vi "Main WT1600 v2.vi"(0 "Settings WT1600 ing":T3={"data bits"=8, "parity"=0, "stop bits"=10, "flow control"=0, "baud rate"=8, "COM"=""} {"baud rate" min=5 max=8 step=1; "flow control" items=["None"=0, "XON/XOFF"=1, "RTS/CTS"=2, "DTR/DSR"=4]; "stop bits" items=["1.0"=10, "1.5"=15, "2.0"=20]; "parity" items=["None", "Odd", "Even", "Mark", "Space"]; "data bits" min=5 max=8 step=1}, 1 "STOP":bool, 2 "Range Tors.":bool, 3 "Numeric":i64, 4 "WT1600 configuration":T2={"Wiring A (0: 1P2W)"=0, "Wiring B (0: 1P2W)"=0, "Wiring C (0: 1P2W)"=0, "V Range (12: 1000)"=12, "Element (0: All)"=0, "Element (0: All) 2"=0, "A Range (9: 5A)"=9, "A Sensor Ratio(mV/A) (10.0000) "=10.0, "Zero Cross Filter (0: OFF)"=0, "Line Filter (0: OFF)"=0, "PT Ratio (1.0000)"=1.0, "Scaling (F: OFF)"=FALSE, "CT Ratio (1.0000)"=1.0, "Scaling Factor (1.0000)"=1.0, "Element (0: All) 3"=0, "Display Format (0: Numeric)"=0, "Normal Item Amount (1: 4)"=1, "Harmonics Item Amount (1: 4)"=1, "Average Type (0: OFF)"=0, "Average Count (2: 8)"=2} {"Average Count (2: 8)" items=["2", "4", "8", "16", "32", "64", "128", "256"]; "Average Type (0: OFF)" items=["OFF", "Linear", "Exponent"]; "Harmonics Item Amount (1: 4)" items=["-", "4", "8", "16", "Single List", "Dual List", "Sigma List"]; "Normal Item Amount (1: 4)" items=["ALL", "4", "8", "16", "42", "78"]; "Display Format (0: Numeric)" items=["Numeric", "Wave", "Bar", "Vector", "Trend", "Numeric & Wave", "Numeric & Bar", "Numeric & Trend", "Wave & Bar", "Wave & Trend", "Bar & Trend", "Information"]; "Element (0: All) 3" items=["All", "Element 1", "Element 2", "Element 3", "Element 4", "Element 5", "Element 6"]; "Scaling Factor (1.0000)" min=0.0001 max=99999.9999 step=0.0001 format="%.4f"; "CT Ratio (1.0000)" min=0.0001 max=99999.9999 step=0.0001 format="%.4f"; "PT Ratio (1.0000)" min=0.0001 max=99999.9999 step=0.0001 format="%.4f"; "Line Filter (0: OFF)" items=["OFF", "500Hz", "5.5kHz"]; "Zero Cross Filter (0: OFF)" items=["OFF", "500Hz"]; "A Sensor Ratio(mV/A) (10.0000)" min=0.0001 max=99999.9999 step=0.0001 format="%.4f"; "A Range (9: 5A)" items=["AUTO", "10 mA", "20 mA", "50 mA", "100 mA", "200 mA", "500 mA", "1 A", "2 A", "5 A", "10 A", "20 A", "50 A", "S-AUTO", "50 mV", "100 mV", "250 mV", "500 mV", "1 V", "2.5 V", "5 V", "10 V"]; "Element (0: All) 2" items=["All", "Element 1", "Element 2", "Element 3", "Element 4", "Element 5", "Element 6"]; "Element (0: All)" items=["All", "Element 1", "Element 2", "Element 3", "Element 4", "Element 5", "Element 6"]; "V Range (12: 1000)" items=["AUTO", "1.5", "3", "6", "10", "15", "30", "60", "100", "150", "300", "600", "1000"]; "Wiring C (0: 1P2W)" items=["1P2W", "1P3W", "3P3W", "3P4W", "3V3A", "NONE"]; "Wiring B (0: 1P2W)" items=["1P2W", "1P3W", "3P3W", "3P4W", "3V3A", "NONE"]; "Wiring A (0: 1P2W)" items=["1P2W", "1P3W", "3P3W", "3P4W", "3V3A"]}, 5 "Refresh":bool, 6 "Clust Refnum":refnum<vi>, 7 "Path":string) -> (9 "error out":errorcluster, 11 "error out 2":errorcluster, 12 "Cluster wt1600":T1, 13 "WT1600 configuration out":T2={"Wiring A (0: 1P2W)"=0, "Wiring B (0: 1P2W)"=0, "Wiring C (0: 1P2W)"=0, "V Range (12: 1000)"=12, "Element (0: All)"=0, "Element (0: All) 2"=0, "A Range (9: 5A)"=9, "A Sensor Ratio(mV/A) (10.0000) "=10.0, "Zero Cross Filter (0: OFF)"=0, "Line Filter (0: OFF)"=0, "PT Ratio (1.0000)"=1.0, "Scaling (F: OFF)"=FALSE, "CT Ratio (1.0000)"=1.0, "Scaling Factor (1.0000)"=1.0, "Element (0: All) 3"=0, "Display Format (0: Numeric)"=0, "Normal Item Amount (1: 4)"=1, "Harmonics Item Amount (1: 4)"=1, "Average Type (0: OFF)"=0, "Average Count (2: 8)"=2} {"Average Count (2: 8)" items=["2", "4", "8", "16", "32", "64", "128", "256"]; "Average Type (0: OFF)" items=["OFF", "Linear", "Exponent"]; "Harmonics Item Amount (1: 4)" items=["-", "4", "8", "16", "Single List", "Dual List", "Sigma List"]; "Normal Item Amount (1: 4)" items=["ALL", "4", "8", "16", "42", "78"]; "Display Format (0: Numeric)" items=["Numeric", "Wave", "Bar", "Vector", "Trend", "Numeric & Wave", "Numeric & Bar", "Numeric & Trend", "Wave & Bar", "Wave & Trend", "Bar & Trend", "Information"]; "Element (0: All) 3" items=["All", "Element 1", "Element 2", "Element 3", "Element 4", "Element 5", "Element 6"]; "Scaling Factor (1.0000)" min=0.0001 max=99999.9999 step=0.0001 format="%.4f"; "CT Ratio (1.0000)" min=0.0001 max=99999.9999 step=0.0001 format="%.4f"; "PT Ratio (1.0000)" min=0.0001 max=99999.9999 step=0.0001 format="%.4f"; "Line Filter (0: OFF)" items=["OFF", "500Hz", "5.5kHz"]; "Zero Cross Filter (0: OFF)" items=["OFF", "500Hz"]; "A Sensor Ratio(mV/A) (10.0000)" min=0.0001 max=99999.9999 step=0.0001 format="%.4f"; "A Range (9: 5A)" items=["AUTO", "10 mA", "20 mA", "50 mA", "100 mA", "200 mA", "500 mA", "1 A", "2 A", "5 A", "10 A", "20 A", "50 A", "S-AUTO", "50 mV", "100 mV", "250 mV", "500 mV", "1 V", "2.5 V", "5 V", "10 V"]; "Element (0: All) 2" items=["All", "Element 1", "Element 2", "Element 3", "Element 4", "Element 5", "Element 6"]; "Element (0: All)" items=["All", "Element 1", "Element 2", "Element 3", "Element 4", "Element 5", "Element 6"]; "V Range (12: 1000)" items=["AUTO", "1.5", "3", "6", "10", "15", "30", "60", "100", "150", "300", "600", "1000"]; "Wiring C (0: 1P2W)" items=["1P2W", "1P3W", "3P3W", "3P4W", "3V3A", "NONE"]; "Wiring B (0: 1P2W)" items=["1P2W", "1P3W", "3P3W", "3P4W", "3V3A", "NONE"]; "Wiring A (0: 1P2W)" items=["1P2W", "1P3W", "3P3W", "3P4W", "3V3A"]}, 14 "Settings WT1600 out":T3={"data bits"=8, "parity"=0, "stop bits"=10, "flow control"=0, "baud rate"=8, "COM"=""} {"baud rate" min=5 max=8 step=1; "flow control" items=["None"=0, "XON/XOFF"=1, "RTS/CTS"=2, "DTR/DSR"=4]; "stop bits" items=["1.0"=10, "1.5"=15, "2.0"=20]; "parity" items=["None", "Odd", "Even", "Mark", "Space"]; "data bits" min=5 max=8 step=1}, 15 "WT1600":bool, 16 "Errori WT1600":i64, 17 "Measure Value":sgl[](array[numeric]) format="%^.3e", 18 "Coppia":dbl, 19 "Velocità":dbl)   [LabVIEW 2016]
uses:
  QSM PC EXAMPLE.llb/wt1600 variabili.ctl
panel:
  in  "termination char\n(0xA = '\\n' = LF)":u8=10 format="%.0x"
  in  "MaxErr WT1600":i64
  # "ON\nOFF"
  # "ON\nOFF"
  # "ON\nOFF"
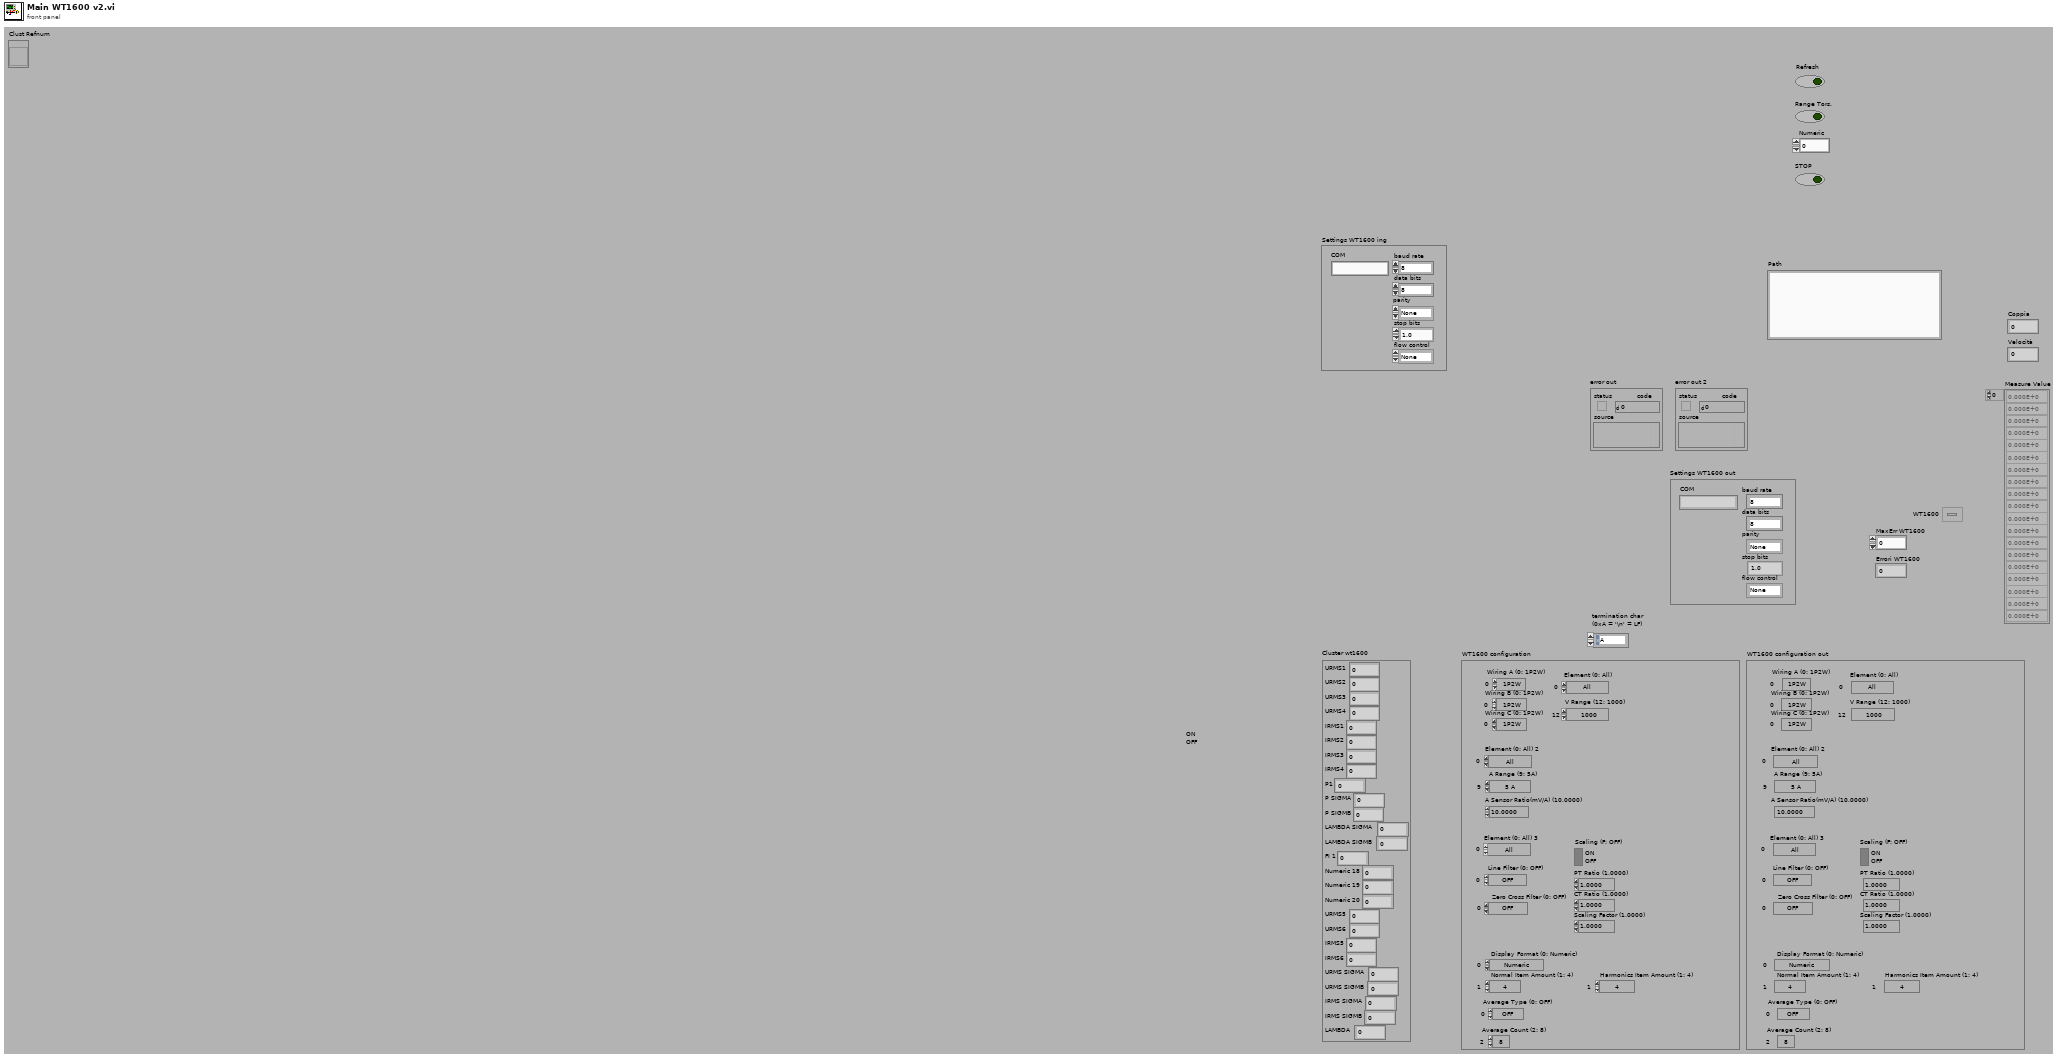
[diagram p1: front panel]
types:
  T1 = typedef "wt1600 variabili.ctl" = cluster{"URMS1":dbl, "URMS2":dbl, "URMS3":dbl, "URMS4":dbl, "IRMS1":dbl, "IRMS2":dbl, "IRMS3":dbl, "IRMS4":dbl, "P1":dbl, "P SIGMA":dbl, "P SIGMB":dbl, "LAMBDA SIGMA":dbl, "LAMBDA SIGMB":dbl, "FI 1":dbl, "Numeric 18":dbl, "Numeric 19":dbl, "Numeric 20":dbl, "URMS5":dbl, "URMS6":dbl, "IRMS5":dbl, "IRMS6":dbl, "URMS SIGMA":dbl, "URMS SIGMB":dbl, "IRMS SIGMA":dbl, "IRMS SIGMB":dbl, "LAMBDA":dbl}
  T2 = cluster{"Wiring A (0: 1P2W)":u16, "Wiring B (0: 1P2W)":u16, "Wiring C (0: 1P2W)":u16, "V Range (12: 1000)":u16, "Element (0: All)":u16, "Element (0: All) 2":u16, "A Range (9: 5A)":u16, "A Sensor Ratio(mV/A) (10.0000) ":dbl, "Zero Cross Filter (0: OFF)":u16, "Line Filter (0: OFF)":u16, "PT Ratio (1.0000)":dbl, "Scaling (F: OFF)":bool, "CT Ratio (1.0000)":dbl, "Scaling Factor (1.0000)":dbl, "Element (0: All) 3":u16, "Display Format (0: Numeric)":u16, "Normal Item Amount (1: 4)":u16, "Harmonics Item Amount (1: 4)":u16, "Average Type (0: OFF)":u16, "Average Count (2: 8)":u16}
  T3 = cluster{"data bits":u16, "parity":u16, "stop bits":u16, "flow control":u16, "baud rate":u16, "COM":string}
  T4 = cluster{"URMS1":dbl, "URMS2":dbl, "URMS3":dbl, "URMS4":dbl, "IRMS1":dbl, "IRMS2":dbl, "IRMS3":dbl, "IRMS4":dbl, "P1":dbl, "P SIGMA":dbl, "P SIGMB":dbl, "LAMBDA SIGMA":dbl, "LAMBDA SIGMB":dbl, "FI 1":dbl, "Numeric 18":dbl, "Numeric 19":dbl, "Numeric 20":dbl, "URMS5":dbl, "URMS6":dbl, "IRMS5":dbl, "IRMS6":dbl, "URMS SIGMA":dbl, "URMS SIGMB":dbl, "IRMS SIGMA":dbl, "IRMS SIGMB":dbl, "LAMBDA":dbl}
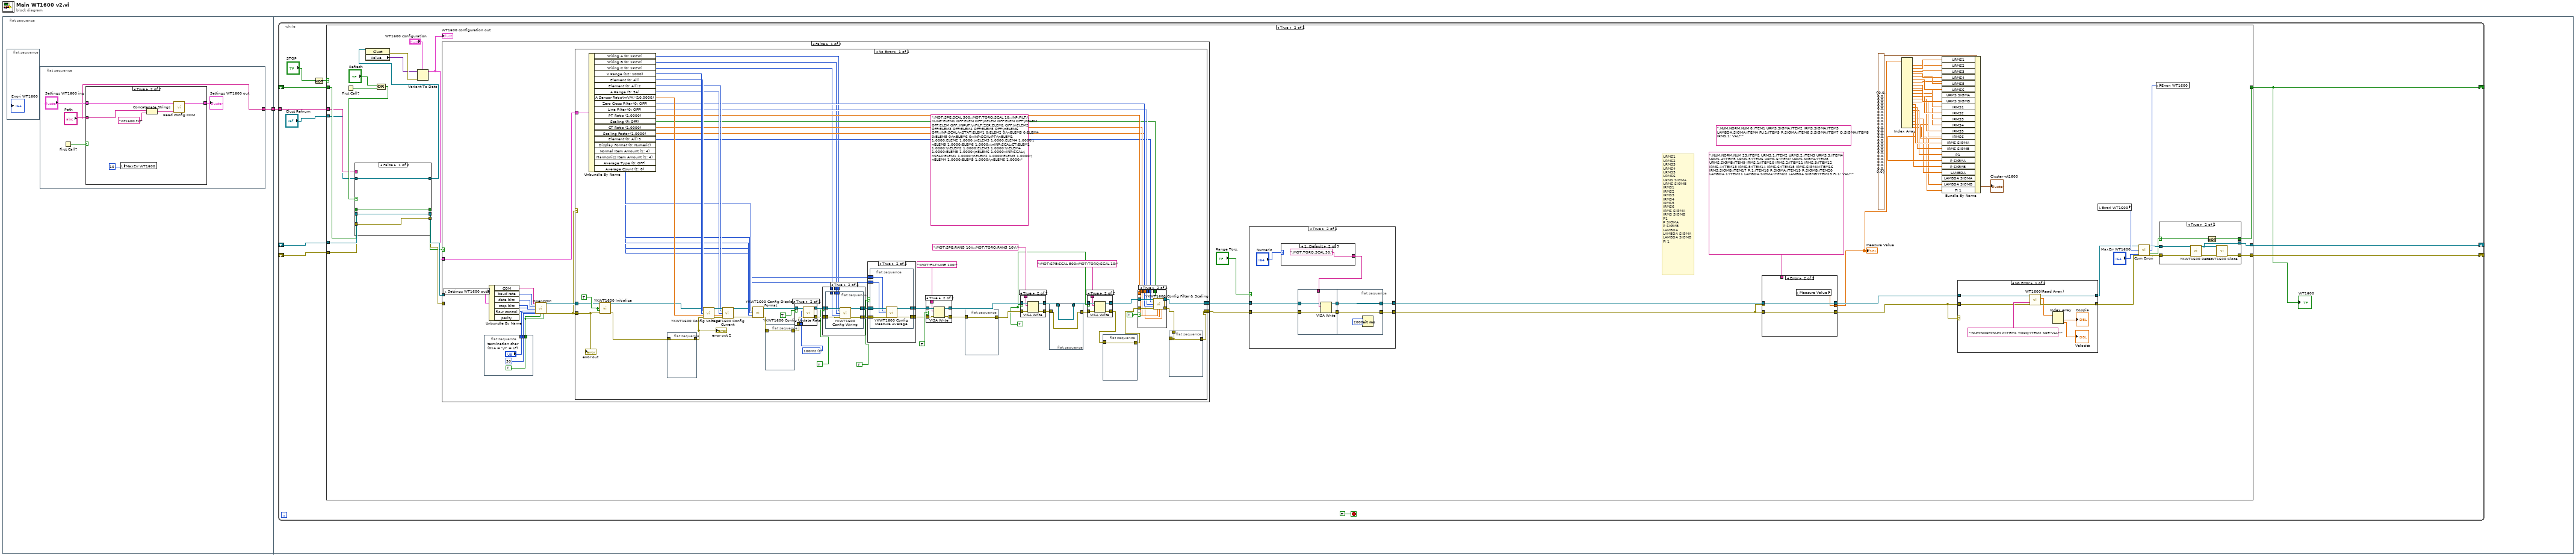
[diagram p0: block diagram]
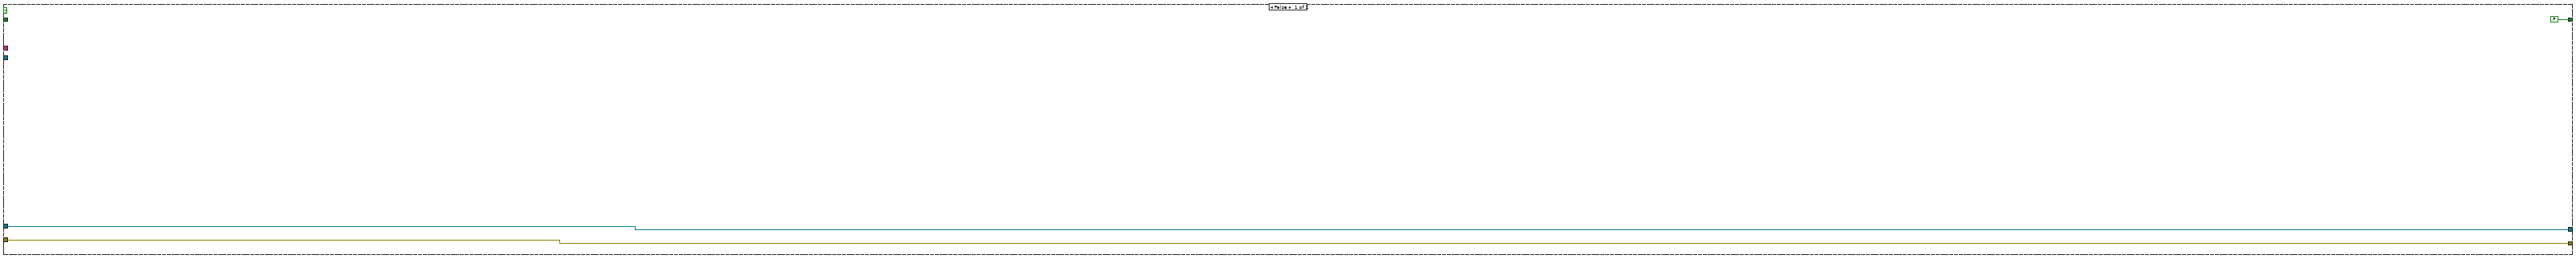
[diagram p3: hidden frame]
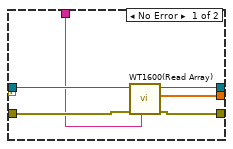
[diagram p4: hidden frame]
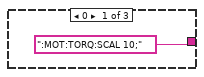
[diagram p6: hidden frame]
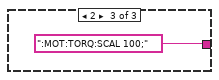
[diagram p7: hidden frame]
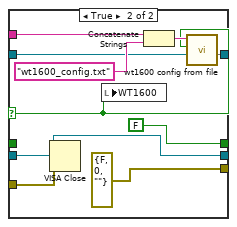
[diagram p9: hidden frame]
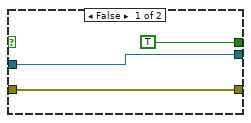
[diagram p19: hidden frame]
diagram:
  n1 = flat-sequence {
    tunnel: [w2] -> w1
    tunnel: w1 -> [w14]
    frame #0 {
      n2 = flat-sequence {
        frame #0 {
        }
      }
      n3 = flat-sequence {
        tunnel: ["Path"] -> w2
        frame #0 {
          n4 = First Call?() -> (First Call?: T/F=w6:bool)
          n5 = case shown="True" w6 {
            tunnel: [w7 w10] -> w4
            tunnel: "Settings WT1600 ing" -> [w7 w11]
            tunnel: "Path" -> [_ w8]
            frame False {
            }
            frame True {
              n6 = local write "MaxErr WT1600"(10) -> ()
              n7 = Concatenate Strings(w8, "wt1600.txt") -> (w12:string)
              n8 = call "Read config COM.vi"("Path"=w12, "Settings WT1600 ing"=w11) -> ("Settings WT1600 out"=w10:T3)  [unwired: 9 out]
            }
          }
          "Settings WT1600 out" <- w4
        }
      }
    }
    frame #1 {
      n9 = while {
        shift-right: [w23] -> _
        shift-left: _ -> [w24]
        shift-right: [w16] -> _
        shift-left: _ -> [w22]
        shift-right: [w15] -> _
        shift-left: _ -> [w25]
        tunnel: w14 -> [w18]
        stop <- TRUE stop-if-true
        n10 = Not(x="STOP") -> (.not. x?=w21:bool)
        n11 = case shown="True" w21 {
          tunnel: w25 -> [_ w79]
          tunnel: w24 -> [w27 w81]
          tunnel: [w27 w89] -> w23
          tunnel: [w28 w88] -> w16
          tunnel: w22 -> [w28 w80]
          tunnel: [FALSE w87] -> w15
          tunnel: w18 -> [_ w69]
          tunnel: "Clust Refnum" -> [_ w63]
          frame False {
          }
          frame True {
            (unwired) ":NUM:NORM:NUM 8;ITEM1 URMS,SIGMA;ITEM2 IRMS,SIGMA;ITEM3 LAMBDA,SIGMA;ITEM4 FU,1;ITEM5 P,SIGMA;ITEM6 S,SIGMA;ITEM7 Q,SIGMA;ITEM8 IRMS,1; VAL?;"
            # "URMS1\nURMS2\nURMS3\nURMS4\nURMS5\nURMS6\nURMS SIGMA\nURMS SIGMB\nIRMS1\nIRMS2\nIRMS3\nIRMS4\nIRMS5\nIRMS6\nIRMS SIGMA\nIRMS SIGMB\nP1\nP SIGMA\nP SIGMB\nLAMBDA\nLAMBDA SIGMA\nLAMBDA SIGMB\nFI 1"
            n12 = First Call?() -> (First Call?: T/F=w72:bool)
            n13 = Compound Arithmetic op=OR("Refresh", w72) -> (w71:bool)
            n14 = case shown="False" w71 {
              selector: w71 -> [_ w137]
              tunnel: [w131 w142] -> w78
              tunnel: w81 -> [w131 w142]
              tunnel: [w132 errorcluster {"status"=FALSE, "code"=0, "source"=""} ("error out")] -> w77
              tunnel: w80 -> [w132 w141]
              tunnel: [w133 FALSE] -> w76
              tunnel: w79 -> [w133 _]
              tunnel: w69 -> [_ w138]
              tunnel: w63 -> [w130 w136]
              tunnel: [w130 w135] -> w62
              frame False {
              }
              frame True {
                n15 = VISA Close(VISA resource name=w142, error in (no error)=w141) -> ()  [unwired: 1 out]
                n16 = local write "WT1600"(w137) -> ()
                n17 = Concatenate Strings(w138, "wt1600_config.txt") -> (w139:string)
                n18 = call "wt1600 config from file.vi"(9:w136, "leggi"=w137, "Path"=w139) -> (1:w135)  [unwired: 1 in, 7 out]
              }
            }
            n19 = property class="Clust"(reference=w62) -> (error out=w68:errorcluster, "Value"=w67:variant)  [unwired: 1 in, 1 out]
            n20 = Variant To Data(error in=w68, type="WT1600 configuration", Variant=w67) -> (data=w60:T2)  [unwired: 1 out]
            "WT1600 configuration out" <- w60
            n21 = case shown="False" w76 {
              tunnel: [w146 w305] -> w64
              tunnel: [w145 w306] -> w65
              tunnel: w77 -> [_ w306]
              tunnel: w78 -> [_ w305]
              tunnel: w60 -> [w149 _]
              frame False {
                n22 = local read "Settings WT1600 out"() -> (w155:T3)
                n23 = flat-sequence {
                  tunnel: [TRUE] -> w158
                  tunnel: ["termination char\n(0xA = '\\n' = LF)"] -> w157
                  tunnel: [50] -> w156
                  frame #0 {
                  }
                }
                n24 = Unbundle By Name(w155) -> ("COM"=w148:string, "baud rate"=w154:u16, "data bits"=w153:u16, "stop bits"=w152:u16, "flow control"=w150:u16, "parity"=w151:u16)
                n25 = call "OpenCOM.vi"("VISA resource name"=w148, "baud rate (9600)"=w154, "data bits"=w153, "parity"=w151, "stop bits"=w152, "flow control"=w150, "termination char\n(0xA = '\\n' = LF)"=w157, "timeout(ms) solitamente 50ms"=w156, "End Write termination character?"=w158, "End read on termination character?"=w158) -> ("VISA resource name out"=w147:refnum<visa-resource-name>, "error out"=w144:errorcluster)  [unwired: 16 out]
                n26 = case shown="No Error" w144 {
                  tunnel: w149 -> [w199 _]
                  tunnel: w144 -> [w196 w301]
                  tunnel: w147 -> [w194 w300]
                  tunnel: [w170 w300] -> w146
                  tunnel: [w165 w301] -> w145
                  frame No Error {
                    w180 = u16 1 items=["50ms", "100ms", "200ms", "500ms", "1s", "2s", "5s"] ("Update Rate (3: 500ms)")
                    (unwired) ":MOT:SPE:SCAL 500;:MOT:TORQ:SCAL 10;:INP:FILT:\nLINE:ELEM1 OFF;ELEM OFF;\nELEM OFF;ELEM OFF;\nELEM OFF;ELEM OFF;:INPUT:\nFILT:ZCR:ELEM1 OFF;\nELEM2 OFF;ELEM3 OFF;ELEM4 OFF;ELEM5 OFF;\nELEM6 OFF;:INP:SCAL:\nSTAT:ELEM1 0;ELEM2 0;\nELEM3 0;ELEM4 0;ELEM5 0;\nELEM6 0;:INP:SCAL:PT:\nELEM1 1.0000;ELEM2 1.0000;\nELEM3 1.0000;ELEM4 1.0000;\nELEM5 1.0000;ELEM6 1.0000;:\nINP:SCAL:CT:ELEM1 1.0000;\nELEM2 1.0000;ELEM3 1.0000;\nELEM4 1.0000;ELEM5 1.0000;\nELEM6 1.0000;:INP:SCAL:\nSFAC:ELEM1 1.0000;\nELEM2 1.0000;ELEM3 1.0000;\nELEM4 1.0000;ELEM5 1.0000;\nELEM6 1.0000;"
                    w176 = TRUE
                    w195 = TRUE
                    n27 = Unbundle By Name(w199) -> ("Wiring A (0: 1P2W)"=w193:u16, "Wiring B (0: 1P2W)"=w192:u16, "Wiring C (0: 1P2W)"=w191:u16, "V Range (12: 1000)"=w219:u16, "Element (0: All)"=w218:u16, "Element (0: All) 2"=w217:u16, "A Range (9: 5A)"=w216:u16, "A Sensor Ratio(mV/A) (10.0000)"=w215:dbl, "Zero Cross Filter (0: OFF)"=w214:u16, "Line Filter (0: OFF)"=w213:u16, "PT Ratio (1.0000)"=w212:dbl, "Scaling (F: OFF)"=w209:bool, "CT Ratio (1.0000)"=w211:dbl, "Scaling Factor (1.0000)"=w210:dbl, "Element (0: All) 3"=w208:u16, "Display Format (0: Numeric)"=w207:u16, "Normal Item Amount (1: 4)"=w206:u16, "Harmonics Item Amount (1: 4)"=w205:u16, "Average Type (0: OFF)"=w201:u16, "Average Count (2: 8)"=w200:u16)
                    n28 = call "YKWT1600 Initialize.vi"("VISA session (for class)"=w194, "ID Query (T: Check)"=w195, "Reset (T: Reset)"=w195, "error in (no error)"=w196) -> ("VISA session"=w160:refnum<visa-resource-name>, "error out"=w159:errorcluster)  [unwired: 10 out]
                    n29 = flat-sequence {
                      tunnel: w159 -> [w222]
                      tunnel: [w222] -> w163
                      frame #0 {
                      }
                    }
                    n30 = call "YKWT1600 Config Voltage.vi"("VISA session"=w160, "Element (0: All)"=w218, "V Range (12: 1000)"=w219, "error in (no error)"=w163) -> ("dup VISA session"=w221:refnum<visa-resource-name>, "error out"=w220:errorcluster)  [unwired: 10 out]
                    n31 = call "YKWT1600 Config Current.vi"("VISA session"=w221, "Element (0: All)"=w217, "A Range (9: 5A)"=w216, 9:w215, "error in (no error)"=w220) -> ("dup VISA session"=w169:refnum<visa-resource-name>, "error out"=w168:errorcluster)  [unwired: 9 out]
                    n32 = call "YKWT1600 Config Display Format.vi"("VISA session"=w169, "Display Format (0: Numeric)"=w207, "Normal Item Amount (1: 4)"=w206, "Harmonics Item Amount (1: 4)"=w205, "error in (no error)"=w168) -> ("dup VISA session"=w184:refnum<visa-resource-name>, "error out"=w185:errorcluster)  [unwired: 9 out]
                    n33 = flat-sequence {
                      tunnel: w185 -> [w271]
                      tunnel: [w271] -> w182
                      frame #0 {
                      }
                    }
                    n34 = case shown="True" TRUE {
                      tunnel: w184 -> [w256 w261]
                      tunnel: [w256 w260] -> w183
                      tunnel: w182 -> [w255 w259]
                      tunnel: [w255 w258] -> w181
                      tunnel: w180 -> [_ w257]
                      frame False {
                      }
                      frame True {
                        n35 = call "YKWT1600 Config Update Rate.vi"("VISA session"=w261, "Update Rate (3: 500ms)"=w257, "error in (no error)"=w259) -> ("dup VISA session"=w260:refnum<visa-resource-name>, "error out"=w258:errorcluster)  [unwired: 11 out]
                      }
                    }
                    n36 = case shown="True" TRUE {
                      tunnel: [w240 w247] -> w203
                      tunnel: [w239 w246] -> w202
                      tunnel: w193 -> [_ w245]
                      tunnel: w192 -> [_ w244]
                      tunnel: w191 -> [_ w243]
                      tunnel: w183 -> [w240 w242]
                      tunnel: w181 -> [w239 w241]
                      frame False {
                      }
                      frame True {
                        n37 = flat-sequence {
                          tunnel: [w253] -> w247
                          tunnel: [w254] -> w246
                          tunnel: w242 -> [w252]
                          tunnel: w241 -> [w251]
                          tunnel: w243 -> [w248]
                          tunnel: w244 -> [w249]
                          tunnel: w245 -> [w250]
                          frame #0 {
                            n38 = call "YKWT1600 Config Wiring.vi"("VISA session"=w252, "Wiring A (0: 1P2W)"=w250, "Wiring B (0: 1P2W)"=w249, "Wiring C (0: 1P2W)"=w248, "error in (no error)"=w251) -> ("dup VISA session"=w253:refnum<visa-resource-name>, "error out"=w254:errorcluster)  [unwired: 9 out]
                          }
                        }
                      }
                    }
                    n39 = case shown="True" TRUE {
                      tunnel: w203 -> [w226 w232]
                      tunnel: w202 -> [w225 w231]
                      tunnel: w201 -> [_ w230]
                      tunnel: w200 -> [_ w229]
                      tunnel: [w226 w228] -> w190
                      tunnel: [w225 w227] -> w172
                      frame False {
                      }
                      frame True {
                        n40 = flat-sequence {
                          tunnel: w232 -> [w238]
                          tunnel: [w237] -> w228
                          tunnel: w231 -> [w236]
                          tunnel: [w235] -> w227
                          tunnel: w230 -> [w234]
                          tunnel: w229 -> [w233]
                          frame #0 {
                            n41 = call "YKWT1600 Config Measure Average.vi"("VISA session"=w238, "Average Type (0: OFF)"=w234, "Average Count (2: 8)"=w233, "error in (no error)"=w236) -> ("dup VISA session"=w237:refnum<visa-resource-name>, "error out"=w235:errorcluster)  [unwired: 10 out]
                          }
                        }
                      }
                    }
                    n42 = case shown="True" TRUE {
                      tunnel: w190 -> [w281 w286]
                      tunnel: w172 -> [w280 w285]
                      tunnel: [w281 w284] -> w198
                      tunnel: [w280 w283] -> w187
                      tunnel: ":MOT:FILT:LINE 100;" -> [_ w282]
                      frame False {
                      }
                      frame True {
                        n43 = VISA Write(VISA resource name=w286, write buffer=w282, error in (no error)=w285) -> (VISA resource name out=w284:refnum<visa-resource-name>, error out=w283:errorcluster)  [unwired: 1 out]
                      }
                    }
                    n44 = flat-sequence {
                      tunnel: w187 -> [w272]
                      tunnel: [w272] -> w186
                      frame #0 {
                      }
                    }
                    n45 = case shown="True" w176 {
                      tunnel: w198 -> [w274 w279]
                      tunnel: w186 -> [w273 w278]
                      tunnel: [w274 w277] -> w162
                      tunnel: [w273 w276] -> w179
                      tunnel: ":MOT:SPE:RANG 10V;:MOT:TORQ:RANG 10V;" -> [_ w275]
                      frame False {
                      }
                      frame True {
                        n46 = VISA Write(VISA resource name=w279, write buffer=w275, error in (no error)=w278) -> (VISA resource name out=w277:refnum<visa-resource-name>, error out=w276:errorcluster)  [unwired: 1 out]
                      }
                    }
                    n47 = flat-sequence {
                      tunnel: w179 -> [w269]
                      tunnel: [w269] -> w177
                      tunnel: w162 -> [w270]
                      tunnel: [w270] -> w161
                      frame #0 {
                      }
                    }
                    n48 = case shown="True" w176 {
                      tunnel: w161 -> [w263 w268]
                      tunnel: w177 -> [w262 w267]
                      tunnel: [w263 w266] -> w171
                      tunnel: [w262 w265] -> w167
                      tunnel: ":MOT:SPE:SCAL 500;:MOT:TORQ:SCAL 10;" -> [_ w264]
                      frame False {
                      }
                      frame True {
                        n49 = VISA Write(VISA resource name=w268, write buffer=w264, error in (no error)=w267) -> (VISA resource name out=w266:refnum<visa-resource-name>, error out=w265:errorcluster)  [unwired: 1 out]
                      }
                    }
                    n50 = flat-sequence {
                      tunnel: w167 -> [w224]
                      tunnel: [w224] -> w164
                      frame #0 {
                      }
                    }
                    n51 = case shown="True" TRUE {
                      tunnel: w171 -> [w288 w299]
                      tunnel: w164 -> [w287 w298]
                      tunnel: w214 -> [_ w297]
                      tunnel: w213 -> [_ w296]
                      tunnel: w212 -> [_ w295]
                      tunnel: w211 -> [_ w294]
                      tunnel: w210 -> [_ w293]
                      tunnel: w209 -> [_ w292]
                      tunnel: w208 -> [_ w291]
                      tunnel: [w288 w290] -> w170
                      tunnel: [w287 w289] -> w166
                      frame False {
                      }
                      frame True {
                        n52 = call "YKWT1600 Config Filter & Scaling.vi"("VISA session"=w299, "Scaling (F: OFF)"=w292, "Element (0: All)"=w291, "Line Filter (0: OFF)"=w296, "WT 1600 Zero Cross Filter (0: OFF)"=w297, "error in (no error)"=w298, "PT Ratio (1.0000)"=w295, "CT Ratio (1.0000)"=w294, "Scaling Factor (1.0000)"=w293) -> ("dup VISA session"=w290:refnum<visa-resource-name>, "error out"=w289:errorcluster)  [unwired: 2 in, 3 out]
                      }
                    }
                    n53 = flat-sequence {
                      tunnel: [w223] -> _
                      tunnel: [w223] -> w165
                      tunnel: w166 -> [w223]
                      frame #0 {
                      }
                    }
                    "error out" <- w196
                    "error out 2" <- w163
                  }
                  frame Error {
                  }
                }
              }
              frame True {
              }
            }
            n54 = case shown="True" "Range Tors." {
              tunnel: w64 -> [w100 w108]
              tunnel: w65 -> [w99 w107]
              tunnel: [w99 w106] -> w30
              tunnel: [w100 w105] -> w59
              frame False {
              }
              frame True {
                n55 = case shown="1, Default" "Numeric" {
                  tunnel: [":MOT:TORQ:SCAL 10;" ":MOT:TORQ:SCAL 50;" ":MOT:TORQ:SCAL 100;"] -> w102
                  frame 0 {
                  }
                  frame 1, Default {
                  }
                  frame 2 {
                  }
                }
                n56 = flat-sequence {
                  tunnel: w102 -> [w116]
                  tunnel: w108 -> [w115]
                  tunnel: w107 -> [w114]
                  tunnel: [w113] -> w104
                  tunnel: [w112] -> w103
                  tunnel: [w118] -> w105
                  tunnel: [w119] -> w106
                  tunnel: w104 -> [w119]
                  tunnel: w103 -> [w118]
                  frame #0 {
                    n57 = VISA Write(VISA resource name=w115, write buffer=w116, error in (no error)=w114) -> (VISA resource name out=w112:refnum<visa-resource-name>, error out=w113:errorcluster)  [unwired: 1 out]
                  }
                  frame #1 {
                    n58 = Wait (ms)(milliseconds to wait=2000) -> ()  [unwired: 1 out]
                  }
                }
              }
            }
            n59 = case shown="Error" w30 {
              tunnel: w30 -> [w95 w97]
              tunnel: w59 -> [w94 w98]
              tunnel: ":NUM:NORM:NUM 23;ITEM1 URMS,1;ITEM2 URMS,2;ITEM3 URMS,3;ITEM4 URMS,4;ITEM5 URMS,5;ITEM6 URMS,6;ITEM7 URMS,SIGMA;ITEM8 URMS,SIGMB;ITEM9 IRMS,1;ITEM10 IRMS,2;ITEM11 IRMS,3;ITEM12 IRMS,4;ITEM13 IRMS,5;ITEM14 IRMS,6;ITEM15 IRMS,SIGMA;ITEM16 IRMS,SIGMB;ITEM17 P,1;ITEM18 P,SIGMA;ITEM19 P,SIGMB;ITEM20 LAMBDA,1;ITEM21 LAMBDA,SIGMA;ITEM22 LAMBDA,SIGMB;ITEM23 FI,1; VAL?;" -> [w93 _]
              tunnel: [w92 w97] -> w29
              tunnel: [w91 w98] -> w57
              tunnel: [w90 w96] -> w41
              frame No Error {
                n60 = call "WT1600(Read Array).vi"("Read"=w93, "error in (no error)"=w95, "VISA session"=w94) -> ("error out"=w92:errorcluster, "Measure 2"=w90:dbl[], "dup VISA session"=w91:refnum<visa-resource-name>)  [unwired: 6 out]
              }
              frame Error {
                n61 = local read "Measure Value"() -> (w96:sgl[])
              }
            }
            "Measure Value" <- w41
            n62 = Index Array(array=w41) -> (element #1=w55:dbl, element #2=w54:dbl, element #3=w53:dbl, element #4=w52:dbl, element #5=w51:dbl, element #6=w50:dbl, element #7=w49:dbl, element #8=w48:dbl, element #9=w47:dbl, element #10=w46:dbl, element #11=w45:dbl, element #12=w44:dbl, element #13=w43:dbl, element #14=w42:dbl, element #15=w40:dbl, element #16=w39:dbl, element #17=w38:dbl, element #18=w37:dbl, element #19=w36:dbl, element #20=w35:dbl, element #21=w34:dbl, element #22=w33:dbl, element #23=w32:dbl)  [unwired: 23 in]
            n63 = Bundle By Name(cluster=T4 {"URMS1"=0.0, "URMS2"=0.0, "URMS3"=0.0, "URMS4"=0.0, "IRMS1"=0.0, "IRMS2"=0.0, "IRMS3"=0.0, "IRMS4"=0.0, "P1"=0.0, "P SIGMA"=0.0, "P SIGMB"=0.0, "LAMBDA SIGMA"=0.0, "LAMBDA SIGMB"=0.0, "FI 1"=0.0, "Numeric 18"=0.0, "Numeric 19"=0.0, "Numeric 20"=0.0, "URMS5"=0.0, "URMS6"=0.0, "IRMS5"=0.0, "IRMS6"=0.0, "URMS SIGMA"=0.0, "URMS SIGMB"=0.0, "IRMS SIGMA"=0.0, "IRMS SIGMB"=0.0, "LAMBDA"=0.0} ("Cluster wt1600"), "URMS1"=w55, "URMS2"=w54, "URMS3"=w53, "URMS4"=w52, "URMS5"=w51, "URMS6"=w50, "URMS SIGMA"=w49, "URMS SIGMB"=w48, "IRMS1"=w47, "IRMS2"=w46, "IRMS3"=w45, "IRMS4"=w44, "IRMS5"=w43, "IRMS6"=w42, "IRMS SIGMA"=w40, "IRMS SIGMB"=w39, "P1"=w38, "P SIGMA"=w37, "P SIGMB"=w36, "LAMBDA"=w35, "LAMBDA SIGMA"=w34, "LAMBDA SIGMB"=w33, "FI 1"=w32) -> (→"Cluster wt1600":T4)
            n64 = case shown="No Error" w29 {
              tunnel: w57 -> [w123 w129]
              tunnel: w29 -> [w122 w128]
              tunnel: [w127 w128] -> w75
              tunnel: [w126 w129] -> w74
              frame No Error {
                n65 = call "WT1600(Read Array).vi"("Read"=":NUM:NORM:NUM 2;ITEM1 TORQ;ITEM2 SPE;VAL?;", "error in (no error)"=w122, "VISA session"=w123) -> ("error out"=w127:errorcluster, "Measure 2"=w125:dbl[], "dup VISA session"=w126:refnum<visa-resource-name>)  [unwired: 6 out]
                n66 = Index Array(array=w125) -> (element #1=→"Coppia":dbl, element #2=→"Velocità":dbl)  [unwired: 2 in]
              }
              frame Error {
              }
            }
            n67 = local read "Errori WT1600"() -> (w84:i64)
            n68 = call "Com Errori.vi"("VISA session"=w74, "Errori in"=w84, "Max Errori"="MaxErr WT1600", "error in (no error)"=w75) -> ("dup VISA session"=w86:refnum<visa-resource-name>, "Errori out"=w83:i64, "Chiudi com"=w61:bool, "error out"=w85:errorcluster)  [unwired: 20 out]
            n69 = local write "Errori WT1600"(w83) -> ()
            n70 = case shown="True" w61 {
              selector: w61 -> [_ w316]
              tunnel: w85 -> [w308 w310]
              tunnel: w86 -> [w309 w313]
              tunnel: [w308 w314] -> w88
              tunnel: [w309 w312] -> w89
              tunnel: [TRUE w315] -> w87
              frame False {
              }
              frame True {
                n71 = call "YKWT1600 Reset.vi"("VISA session"=w313, "error in (no error)"=w310) -> ("dup VISA session"=w312:refnum<visa-resource-name>, "error out"=w311:errorcluster)  [unwired: 12 out]
                n72 = Not(x=w316) -> (.not. x?=w315:bool)
                n73 = call "YKWT1600 Close.vi"("VISA session"=w312, "error in (no error)"=w311) -> ("error out"=w314:errorcluster)  [unwired: 13 out]
              }
            }
          }
        }
        "WT1600" <- w15
      }
    }
  }
